vi "Secure-Release Region.vi"(7 "Action":enum16{"Secure", "Release"}(ring), 8 "error in (no error)":errorcluster, 10 "Control In":T1, 11 "Carrier Tray in":refnum<class "Assembly Tray.lvclass">) -> (0 "error out":errorcluster, 2 "Control Out":T1, 3 "Carrier Tray out":refnum<class "Assembly Tray.lvclass">)   [LabVIEW 2020, in "Assembly Tray.lvclass"]
uses:
  Assembly Tray.lvclass
  C:/Users/hep/Documents/CMU gantry/Classes/Workspace/Fixture.lvclass
  Controller/Controllers.ctl
  Controller/I-O/I-O.lvclass
  Controller/Dispenser/Dispenser.lvclass
  C:/Program Files (x86)/Aerotech/A3200/LabVIEW/2010/Bin/Aerotech.A3200.dll
  Program Files (x86)/Aerotech/A3200/LabVIEW/2010/Bin/Aerotech.A3200.dll
  Fixture.lvclass/Fixture.ctl
  Assembly Tray.lvclass/Assembly Tray.ctl
  Fixture.lvclass
  Controller/Controller.lvclass
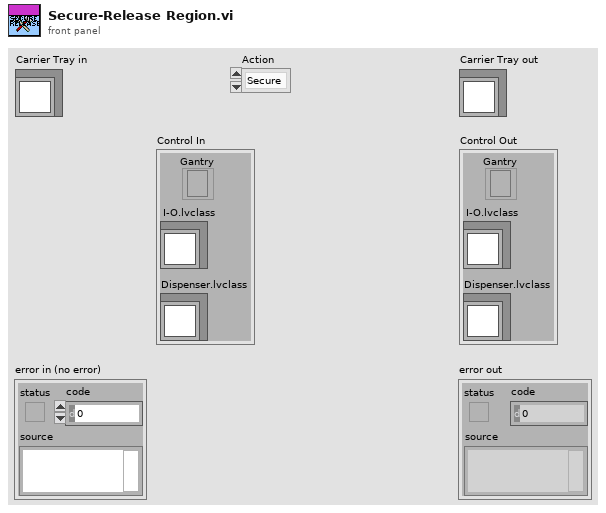
[diagram p1: front panel]
types:
  T1 = typedef "Controller.lvclass/Controllers.ctl" = cluster{"I-O.lvclass":refnum<class "I-O.lvclass">, "Dispenser.lvclass":refnum<class "Dispenser.lvclass">, "Gantry":refnum<k24>}
  T2 = typedef "I-O.lvclass/Pin Map.ctl" = cluster{"Region Valves":i32[], "Extra Valves":dbl[][][], "Tool Primary Valve":i32, "Tool Secondary Valve":i32, "Region Sensors":i32[], "Extra Sensors":dbl[][][], "Tool Primary Sensor":dbl, "Tool Secondary Sensor":dbl, "Compression Sensor":dbl, "5V":i32}
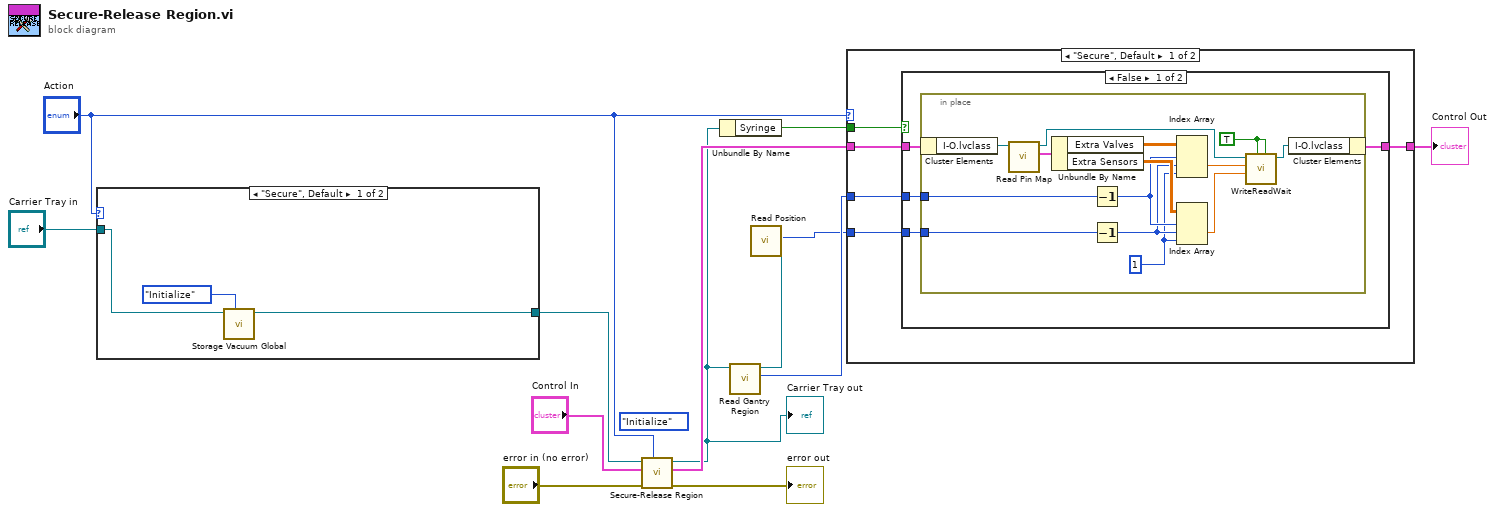
[diagram p0: block diagram]
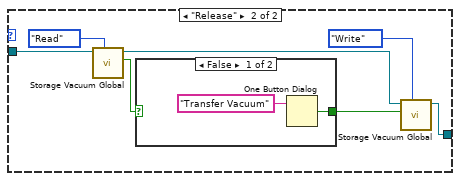
[diagram p4: hidden frame]
diagram:
  (unwired) enum16{"Initialize", "Read", "Write"}."Initialize" ("Action")
  n1 = case shown="\"Secure\", Default" "Action" {
    tunnel: [w15 w18] -> w10
    tunnel: "Carrier Tray in" -> [w14 w17]
    frame "Secure", Default {
      n2 = call "Storage Vacuum Global.vi"("Action"=enum16{"Initialize", "Read", "Write"}."Initialize", "Carrier Tray.lvclass"=w14) -> ("Carrier Tray.lvclass 2"=w15:refnum<class "Assembly Tray.lvclass">)  [unwired: 7 in, 2 out]
    }
    frame "Release" {
      n3 = call "Storage Vacuum Global.vi"("Action"=enum16{"Initialize", "Read", "Write"}."Read", "Carrier Tray.lvclass"=w17) -> ("Read"=w23:bool, "Carrier Tray.lvclass 2"=w19:refnum<class "Assembly Tray.lvclass">)  [unwired: 7 in, 1 out]
      n4 = case shown="False" w23 {
        selector: w23 -> [_ w26]
        tunnel: [w24 w26] -> w20
        frame False {
          n5 = One Button Dialog(message="Transfer Vacuum") -> (true=w24:bool)  [unwired: 1 in]
        }
        frame True {
        }
      }
      n6 = call "Storage Vacuum Global.vi"("Action"=enum16{"Initialize", "Read", "Write"}."Write", "Write"=w20, "Carrier Tray.lvclass"=w19) -> ("Carrier Tray.lvclass 2"=w18:refnum<class "Assembly Tray.lvclass">)  [unwired: 6 in, 2 out]
    }
  }
  n7 = call-parent "Secure-Release Region.vi"("Action"="Action", "error in (no error)"="error in (no error)", "Control In"="Control In", "Fixture in"=w10) -> ("error out"=→"error out":errorcluster, "Control Out"=w8:T1, "Fixture out"=w1:refnum<class "Assembly Tray.lvclass">)  [unwired: 5 in]
  "Carrier Tray out" <- w1
  n8 = Unbundle By Name(w1) -> ("Syringe"=w9:bool)
  n9 = call "Read Gantry Region.vi"("Fixture in"=w1) -> ("Gantry Region"=w6:i32, "Fixture out"=w7:refnum<class "Assembly Tray.lvclass">)  [unwired: 8 in, 1 out]
  n10 = call "Read Position.vi"("Fixture in"=w7) -> ("Position"=w5:i32)  [unwired: 8 in, 2 out]
  n11 = case shown="\"Secure\", Default" "Action" {
    tunnel: w9 -> [w31 _]
    tunnel: w8 -> [w30 w51]
    tunnel: w6 -> [w29 _]
    tunnel: w5 -> [w28 _]
    tunnel: [w27 w51] -> w4
    frame "Secure", Default {
      n12 = case shown="False" w31 {
        tunnel: w30 -> [w35 w50]
        tunnel: w29 -> [w34 _]
        tunnel: w28 -> [w33 _]
        tunnel: [w32 w50] -> w27
        frame False {
          n13 = in-place {
            in-place-border: w34 -> [w43]
            in-place-border: w33 -> [w41]
            w39 = 1
            w45 = TRUE
            n14 = in-place-cluster #1(w35) -> ("I-O.lvclass"=w49:refnum<class "I-O.lvclass">)
            n15 = call-dynamic "Read Pin Map.vi"("I-O in"=w49) -> ("Pin Map 2"=w48:T2, "I-O out"=w46:refnum<class "I-O.lvclass">)  [unwired: 8 in, 1 out]
            n16 = Unbundle By Name(w48) -> ("Extra Valves"=w36:dbl[][][], "Extra Sensors"=w47:dbl[][][])
            n17 = Decrement(x=w43) -> (x-1=w42:i32)
            n18 = Decrement(x=w41) -> (x-1=w40:i32)
            n19 = Index Array(array=w36, index (dim 0)=w42, index (dim 1)=w40, index (dim 2)=w39) -> (element=w38:dbl)
            n20 = Index Array(array=w47, index (dim 0)=w42, index (dim 1)=w40, index (dim 2)=w39) -> (element=w37:dbl)
            n21 = call "WriteReadWait.vi"("Read Value"=w45, "Write Value"=w45, "Read"=w37, "Write"=w38, "I-O in"=w46) -> ("I-O out"=w44:refnum<class "I-O.lvclass">)  [unwired: 5 in, 1 out]
            n22 = in-place-cluster #1("I-O.lvclass"=w44) -> (w32:T1)
          }
        }
        frame True {
        }
      }
    }
    frame "Release" {
    }
  }
  "Control Out" <- w4
